vi "MultiScanDrift_dev_multiparam.vi"() -> ()   [LabVIEW 2014]
uses:
  shared/CorrelImages (SubVI)Single.vi
  <userlib>/Nanonis Prog Interface V5/Nanonis Prog Interface.lvlib
panel:
  out "size(s)":i32
  in  "max steps":i32
  in  "Lockin ON/OFF":bool
  in  "Multipass":bool=TRUE
  in  "Add":bool
  in  "end":sgl=1.0 format="%#_6p"
  in  "step":sgl=0.05 format="%#_6p"
  in  "start":sgl=-1.5 format="%#_6p"
  in  "create Range":bool
  in  "PLL ON/OFF":bool
  in  "ref bias":dbl=-0.0012 format="%#_6p"
  in  "ref setpoint":bool
  in  "DC On":bool=TRUE
  out "Y drift":i32
  out "X drift":i32
  out "DC active":bool
  in  "Drift correction Pixels":i32=128
  in  "Img Current":sgl=1e-10 format="%#_6p"
  in  "Img Bias (V) DC":sgl=1.0 format="%_2p"
  in  "Forward Speed":sgl=1.2e-09 format="%#_6p"
  in  "Backward Speed":sgl=8e-08 format="%#_6p"
  in  "Img Speed":sgl=4.5e-08 format="%#_6p"
  in  "Channel index (0-23)":u8(ring) items=["Current"=0, "Z (m)"=14]
  in  "Settling time (s)":dbl=0.7 format="%#_6p"
  in  "img bias":bool
  in  "img bias":dbl=-0.0012 format="%#_6p"
  in  "img delay (s)":u32=1
  out "Bias_mod":dbl format="%#_6p"
  in  "Bias_mod List":i32(listbox)
  in  "Const Height":bool
  in  "CurrentList":i32(listbox)
  in  "BiasList":i32(listbox)=35
  out "Current":dbl=5e-11 format="%#_6p"
  out "Bias":dbl=0.02 format="%#_6p"
  # "- Do Not Use This unless you are planning to change Lockin Amplitude for each bias. \n- This version will run experiments with parameters specified in each line."
  # "Turn continuous scan off\n zero tiplift is '0'"
  # "Multipass Windows \nneeds to be open\n and OFF"
  # "5"
  # "10"
  # "15"
  # "20"
  # "25"
  # "30"
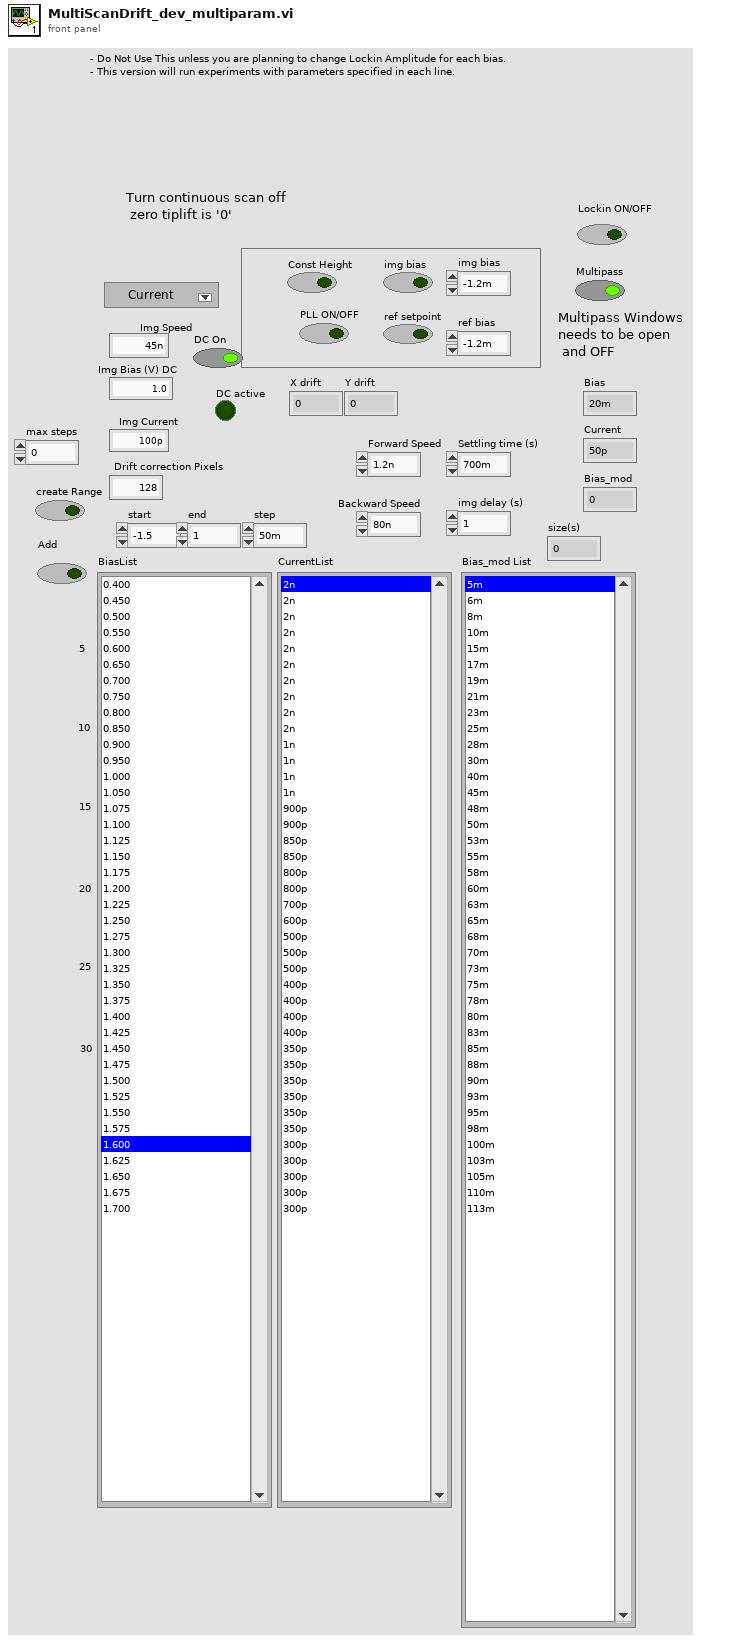
[diagram p1: front panel]
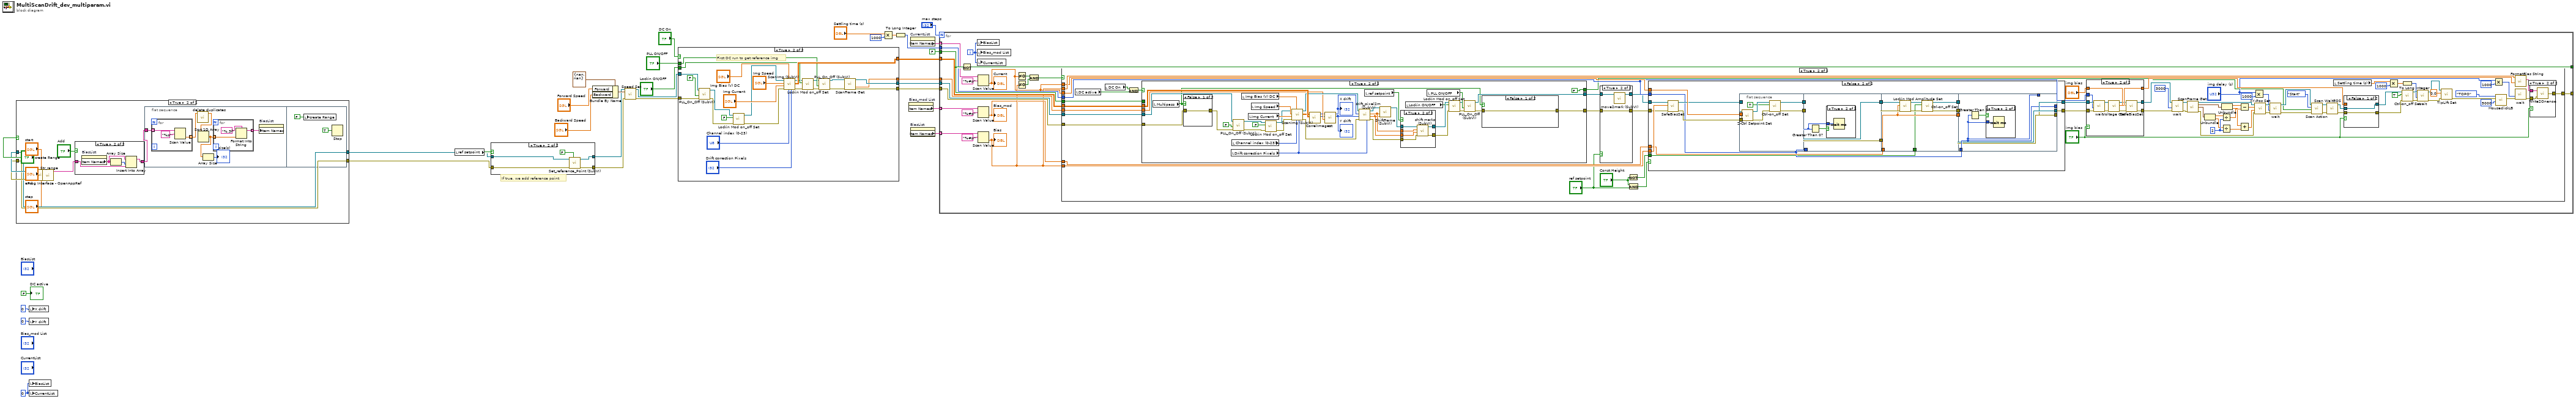
[diagram p0: block diagram]
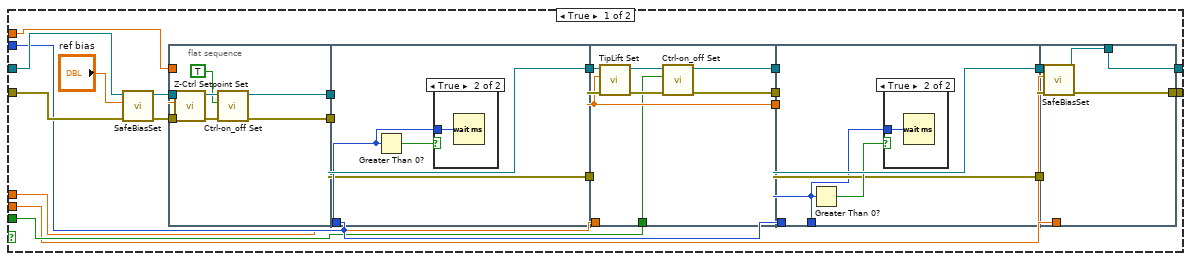
[diagram p4: hidden frame]
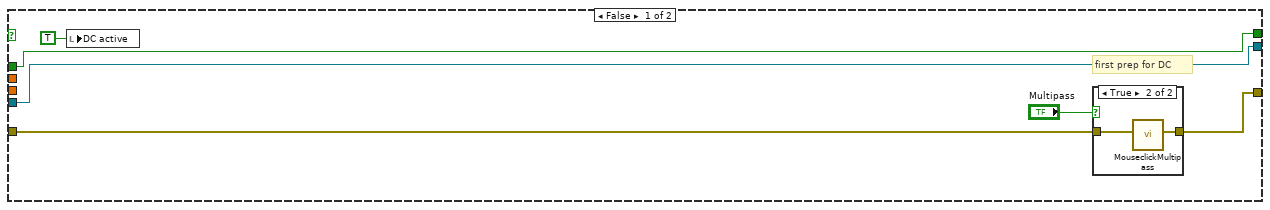
[diagram p10: hidden frame]
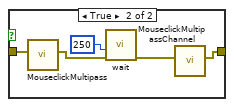
[diagram p13: hidden frame]
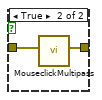
[diagram p14: hidden frame]
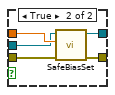
[diagram p15: hidden frame]
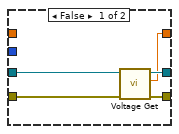
[diagram p16: hidden frame]
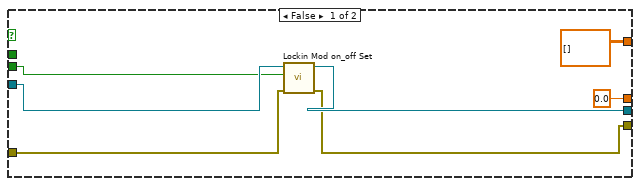
[diagram p20: hidden frame]
diagram:
  w34 = 0 ("BiasList")
  # "If true, we add reference point"
  n1 = local write "X drift"(0 ("X drift")) -> ()
  n2 = local write "Y drift"(0 ("Y drift")) -> ()
  n3 = local write "BiasList"(w34) -> ()
  n4 = local write "CurrentList"(w34) -> ()
  n5 = call <userlib>:"Prog Interface - OpenAppRef.vi"() -> ("Error out"=w9:errorcluster, "Application reference"=w10:refnum<vi>)  [unwired: 6 in]
  n6 = case shown="True" "create Range" {
    tunnel: w10 -> [w36 w44]
    tunnel: [w36 w44] -> w5
    tunnel: w9 -> [w35 w43]
    tunnel: [w35 w43] -> w7
    frame False {
    }
    frame True {
      n7 = call "Str_range.vi"("step"="step", "end"="end", "start"="start") -> ("Item Names"=w37:string[])  [unwired: 8 in]
      n8 = case shown="True" "Add" {
        tunnel: [w59 w61] -> w38
        tunnel: w37 -> [w59 w60]
        frame False {
        }
        frame True {
          n9 = property on="BiasList" class="LstBox (strict)"() -> ("Item Names"=w62:string[])  [unwired: 2 in, 2 out]
          n10 = Array Size(array=w62) -> (size(s)=w63:i32)
          n11 = Insert Into Array(array=w62, index=w63, new element=w60) -> (w61:string[])
        }
      }
      n12 = flat-sequence {
        tunnel: w38 -> [w50]
        frame #0 {
          n13 = for {
            tunnel: w50 -> [w56] mode=indexing
            tunnel: [w54] -> w46 mode=indexing
            n14 = Scan Value(string=w56, format string="%p") -> (value=w54:dbl)  [unwired: 1 in, 1 out]
          }
          n15 = call "delete duplicates.vi"("Array"=w46) -> ("Output array"=w45:dbl[])  [unwired: 10 in]
          n16 = Sort 1D Array(array=w45) -> (sorted array=w48:dbl[])
          n17 = Array Size(array=w48) -> (size(s)=→"size(s)":i32)
          n18 = for {
            tunnel: w48 -> [w53] mode=indexing
            tunnel: [w52] -> w49 mode=indexing
            n19 = Format Into String(format string="%.3f", w53) -> (resulting string=w52:string)  [unwired: 2 in, 1 out]
          }
          n20 = property on="BiasList" class="LstBox (strict)"("Item Names"=w49) -> ()  [unwired: 2 in, 2 out]
        }
        frame #1 {
          n21 = local write "create Range"(FALSE ("Range")) -> ()
          n22 = Stop(stop? (T)=TRUE) -> ()
        }
      }
    }
  }
  n23 = local read "ref setpoint"() -> (w8:bool)
  n24 = case shown="True" w8 {
    tunnel: w7 -> [w65 w69]
    tunnel: [w65 w68] -> w6
    tunnel: w5 -> [w64 w67]
    tunnel: [w64 w66] -> w4
    frame False {
    }
    frame True {
      n25 = call "Set_reference_Point (SubVI).vi"("Part of multigrid"=FALSE, "error in (no error)"=w69, "Application in"=w67) -> ("error out"=w68:errorcluster, "Application out"=w66:refnum<vi>)  [unwired: 7 in]
    }
  }
  n26 = Bundle By Name(cluster=cluster{"Forward":sgl, "Backward":sgl} {"Forward"=nan, "Backward"=nan} ("Speed (m/s)"), "Forward"="Forward Speed", "Backward"="Backward Speed") -> (w21:cluster{"Forward":sgl, "Backward":sgl})
  n27 = call <userlib>:"Speed Set.vi"("Application ref in"=w4, "Speed (m/s)"=w21, "error in (no error)"=w6) -> ("Application ref out"=w19:refnum<vi>, "error out"=w18:errorcluster)  [unwired: 11 in]
  n28 = case shown="True" "DC On" {
    tunnel: [w74 w91] -> w23
    tunnel: [w72 w90] -> w22
    tunnel: [dbl[][] [] ("Img") w98] -> w20
    tunnel: w19 -> [w75 w97]
    tunnel: w18 -> [w73 w96]
    tunnel: [sgl 0.0 ("Angle (deg)") w89] -> w13
    tunnel: "PLL ON/OFF" -> [_ w88]
    tunnel: "Lockin ON/OFF" -> [w71 w82]
    frame False {
      n29 = call <userlib>:"Lockin Mod on_off Set.vi"("Error in (no error)"=w73, "Lockin ON/OFF"=w71, "Application ref in"=w75) -> ("Error out"=w72:errorcluster, "Application ref out"=w74:refnum<vi>)  [unwired: 7 in]
    }
    frame True {
      # "First DC run to get reference img"
      n30 = call "PLL_On_Off (SubVI).vi"("error in (no error)"=w96, "Output ON/OFF (F=OFF)"=FALSE, "Application in"=w97) -> ("error out"=w85:errorcluster, "Application out"=w86:refnum<vi>)  [unwired: 7 in]
      n31 = call <userlib>:"Lockin Mod on_off Set.vi"("Error in (no error)"=w85, "Lockin ON/OFF"=FALSE, "Application ref in"=w86) -> ("Error out"=w84:errorcluster, "Application ref out"=w83:refnum<vi>)  [unwired: 7 in]
      n32 = call "ScanImg (SubVI).vi"("pixel"="Drift correction Pixels", "Channel index (0-23)"="Channel index (0-23)", "Bias (V)"="Img Bias (V) DC", "error in (no error)"=w84, "Current"="Img Current", "Img Speed"="Img Speed", "Application in"=w83) -> ("error out"=w79:errorcluster, "Img"=w98:dbl[][], "Application out"=w81:refnum<vi>)  [unwired: 2 in]
      n33 = call <userlib>:"Lockin Mod on_off Set.vi"("Error in (no error)"=w79, "Lockin ON/OFF"=w82, "Application ref in"=w81) -> ("Error out"=w78:errorcluster, "Application ref out"=w80:refnum<vi>)  [unwired: 7 in]
      n34 = call "PLL_On_Off (SubVI).vi"("error in (no error)"=w78, "Output ON/OFF (F=OFF)"=w88, "Application in"=w80) -> ("error out"=w92:errorcluster, "Application out"=w93:refnum<vi>)  [unwired: 7 in]
      n35 = call <userlib>:"ScanFrame Get.vi"("Application ref in"=w93, "error in (no error)"=w92) -> ("Application ref out"=w91:refnum<vi>, "Angle (deg)"=w89:sgl, "error out"=w90:errorcluster)  [unwired: 9 in, 2 out]
    }
  }
  n36 = Multiply(x="Settling time (s)", y=u32 1000) -> (x*y=w30:dbl)
  n37 = To Long Integer(number=w30) -> (32bit integer=w31:i32)
  n38 = property on="Bias_mod List" class="LstBox (strict)"() -> ("Item Names"=w2:string[])  [unwired: 2 in, 2 out]
  n39 = property on="CurrentList" class="LstBox (strict)"() -> ("Item Names"=w27:string[])  [unwired: 2 in, 2 out]
  n40 = property on="BiasList" class="LstBox (strict)"() -> ("Item Names"=w28:string[])  [unwired: 2 in, 2 out]
  n41 = for {
    N: "max steps" -> [_]
    tunnel: w28 -> [w118] mode=indexing
    tunnel: w23 -> [w120]
    tunnel: w22 -> [w119]
    tunnel: FALSE ("Direction: up/down (T=up)") -> [w122]
    tunnel: [w121] -> _
    tunnel: w31 -> [w114]
    tunnel: w20 -> [w113]
    tunnel: w13 -> [w112]
    tunnel: [w110] -> _
    tunnel: w27 -> [w107] mode=indexing
    tunnel: w2 -> [w106] mode=indexing
    i -> [w103]
    n42 = Not(x=w122) -> (.not. x?=w121:bool)
    n43 = local write "BiasList"(w103) -> ()
    n44 = local write "Bias_mod List"(w103) -> ()
    n45 = local write "CurrentList"(w103) -> ()
    n46 = Scan Value(string=w107, format string="%#p") -> (value=w105:dbl)  [unwired: 1 in, 1 out]
    "Current" <- w105
    n47 = Scan Value(string=w106, format string="%#p") -> (value=w104:dbl)  [unwired: 1 in, 1 out]
    "Bias_mod" <- w104
    n48 = Scan Value(string=w118, format string="%#p") -> (value=w111:dbl)  [unwired: 1 in, 1 out]
    "Bias" <- w111
    n49 = Not Equal To 0?(x=w105) -> (x != 0?=w117:bool)
    n50 = Not Equal To 0?(x=w111) -> (x != 0?=w116:bool)
    n51 = Compound Arithmetic op=AND(w117, w116) -> (w115:bool)
    n52 = case shown="True" w115 {
      tunnel: w122 -> [_ w176]
      tunnel: w111 -> [_ w202]
      tunnel: w120 -> [_ w181]
      tunnel: w119 -> [w124 w180]
      tunnel: w105 -> [_ w203]
      tunnel: w104 -> [_ w199]
      tunnel: w114 -> [_ w183]
      tunnel: w113 -> [_ w182]
      tunnel: w112 -> [_ w175]
      tunnel: w111 -> [_ w174]
      tunnel: w105 -> [_ w173]
      tunnel: [w124 w169] -> w110
      frame False {
      }
      frame True {
        w155 = 2
        n53 = local read "DC active"() -> (w179:bool)
        n54 = local read "DC On"() -> (w178:bool)
        n55 = And(x=w178, y=w179) -> (x .and. y?=w177:bool)
        n56 = case shown="True" w177 {
          tunnel: w182 -> [_ w357]
          tunnel: w181 -> [w314 w349]
          tunnel: w180 -> [w310 w338]
          tunnel: [w309 w334] -> w135
          tunnel: [w314 w348] -> w136
          tunnel: [w312 FALSE ("Direction: up/down (T=up)")] -> w140
          tunnel: w176 -> [w312 _]
          tunnel: w175 -> [_ w344]
          frame False {
            # "first prep for DC"
            n57 = local write "DC active"(TRUE ("DC active")) -> ()
            n58 = case shown="True" "Multipass" {
              tunnel: w310 -> [w315 w317]
              tunnel: [w315 w316] -> w309
              frame False {
              }
              frame True {
                n59 = call "MouseclickMultipass.vi"("error in (no error)"=w317) -> ("error out"=w316:errorcluster)  [unwired: 10 in]
              }
            }
          }
          frame True {
            n60 = local read "Multipass"() -> (w333:bool)
            n61 = case shown="False" w333 {
              tunnel: w338 -> [w372 w374]
              tunnel: [w372 w373] -> w337
              frame False {
              }
              frame True {
                n62 = call "MouseclickMultipass.vi"("error in (no error)"=w374) -> ("error out"=w373:errorcluster)  [unwired: 10 in]
              }
            }
            n63 = local read "Drift correction Pixels"() -> (w346:i32)
            n64 = local read "Channel index (0-23)"() -> (w352:u8)
            n65 = call "PLL_On_Off (SubVI).vi"("error in (no error)"=w337, "Output ON/OFF (F=OFF)"=FALSE, "Application in"=w349) -> ("error out"=w327:errorcluster, "Application out"=w325:refnum<vi>)  [unwired: 7 in]
            n66 = local read "Img Bias (V) DC"() -> (w353:sgl)
            n67 = local read "Img Current"() -> (w354:sgl)
            n68 = local read "Img Speed"() -> (w355:sgl)
            n69 = call <userlib>:"Lockin Mod on_off Set.vi"("Error in (no error)"=w327, "Lockin ON/OFF"=FALSE, "Application ref in"=w325) -> ("Error out"=w326:errorcluster, "Application ref out"=w324:refnum<vi>)  [unwired: 7 in]
            n70 = call "ScanImg (SubVI).vi"("pixel"=w346, "Channel index (0-23)"=w352, "Bias (V)"=w353, "error in (no error)"=w326, "Current"=w354, "Img Speed"=w355, "Application in"=w324) -> ("error out"=w336:errorcluster, "Img"=w356:dbl[][], "Application out"=w350:refnum<vi>)  [unwired: 2 in]
            n71 = call-poly "CorrelImages.vi"("Ref Array"=w357, "New Image"=w356) -> ("Y drift"=w341:i32, "X drift"=w343:i32)  [unwired: 6 in, 2 out]
            n72 = call "rot.vi"("angle"=w344, "y"=w341, "x"=w343) -> ("y'"=w340:i32, "x'"=w342:i32)  [unwired: 7 in]
            "X drift" <- w342
            "Y drift" <- w340
            n73 = call "drift_pixel2m (SubVI).vi"("Application in"=w350, "X drift"=w342, "Y drift"=w340, "error in"=w336, "Drift correction Pixels"=w346) -> ("Application out"=w351:refnum<vi>, "x drift"=w331:sgl, "y drift"=w330:sgl, "error out"=w329:errorcluster)  [unwired: 1 in]
            n74 = local read "ref setpoint"() -> (w332:bool)
            n75 = call "ShiftFrame (SubVI).vi"("Y shift"=w330, "X shift"=w331, "Application in"=w351) -> ("Application out"=w328:refnum<vi>)  [unwired: 8 in]
            n76 = case shown="True" w332 {
              tunnel: w331 -> [_ w365]
              tunnel: w330 -> [_ w364]
              tunnel: w329 -> [w358 w363]
              tunnel: [w358 w362] -> w320
              tunnel: w328 -> [w359 w361]
              tunnel: [w359 w360] -> w319
              frame False {
              }
              frame True {
                n77 = call "shift marks (SubVI).vi"("error in (no error)"=w363, "y"=w364, "x"=w365, "Application in"=w361) -> ("error out"=w362:errorcluster, "Application out"=w360:refnum<vi>)  [unwired: 6 in]
              }
            }
            n78 = local read "Lockin ON/OFF"() -> (w318:bool)
            n79 = local read "PLL ON/OFF"() -> (w339:bool)
            n80 = call <userlib>:"Lockin Mod on_off Set.vi"("Error in (no error)"=w320, "Lockin ON/OFF"=w318, "Application ref in"=w319) -> ("Error out"=w321:errorcluster, "Application ref out"=w322:refnum<vi>)  [unwired: 7 in]
            n81 = call "PLL_On_Off (SubVI).vi"("error in (no error)"=w321, "Output ON/OFF (F=OFF)"=w339, "Application in"=w322) -> ("error out"=w335:errorcluster, "Application out"=w348:refnum<vi>)  [unwired: 7 in]
            n82 = case shown="False" w333 {
              tunnel: w335 -> [w366 w371]
              tunnel: [w366 w370] -> w334
              frame False {
              }
              frame True {
                n83 = call "MouseclickMultipass.vi"("error in (no error)"=w371) -> ("error out"=w369:errorcluster)  [unwired: 10 in]
                n84 = call "wait.vi"("error in"=w369, "milliseconds to wait"=u32 250) -> ("error out"=w368:errorcluster)  [unwired: 8 in, 1 out]
                n85 = call "MouseclickMultipassChannel.vi"("error in (no error)"=w368) -> ("error out"=w370:errorcluster)  [unwired: 10 in]
              }
            }
          }
        }
        n86 = case shown="True" "ref setpoint" {
          tunnel: w136 -> [w205 w208]
          tunnel: w135 -> [w204 w207]
          tunnel: [w204 w207] -> w133
          tunnel: [w205 w206] -> w134
          frame False {
          }
          frame True {
            n87 = call "move2mark (SubVI).vi"("Application in"=w208) -> ("Application out"=w206:refnum<vi>)  [unwired: 10 in]
          }
        }
        n88 = Not(x="Const Height") -> (.not. x?=w201:bool)
        n89 = And(x="Const Height", y="ref setpoint") -> (x .and. y?=w167:bool)
        n90 = case shown="False" w167 {
          tunnel: w203 -> [w216 w268]
          tunnel: w202 -> [w211 w278]
          tunnel: w201 -> [w212 w263]
          tunnel: w199 -> [w213 w265]
          tunnel: [w210 w262] -> w196
          tunnel: [w209 w261] -> w195
          tunnel: w183 -> [w217 w264]
          tunnel: w133 -> [w227 w277]
          tunnel: w134 -> [w228 w276]
          frame True {
            n91 = call "SafeBiasSet.vi"("Application ref in"=w228, "Bias (V)"="ref bias", "error in (no error)"=w227) -> ("Application ref out"=w215:refnum<vi>, "Error out"=w214:errorcluster)  [unwired: 6 in]
            n92 = flat-sequence {
              tunnel: [w236] -> w226
              tunnel: [w233] -> w225
              tunnel: w216 -> [w232]
              tunnel: w215 -> [w231]
              tunnel: w214 -> [w230]
              tunnel: w226 -> [w241]
              tunnel: [w241] -> w224
              tunnel: w217 -> [w239]
              tunnel: [w238] -> w223
              tunnel: w225 -> [w238]
              tunnel: w224 -> [w250]
              tunnel: [w248] -> w222
              tunnel: [w244] -> w221
              tunnel: w223 -> [w247]
              tunnel: [w245] -> w220
              tunnel: w213 -> [w244]
              tunnel: w212 -> [w243]
              tunnel: w222 -> [w254]
              tunnel: [w251] -> _
              tunnel: w221 -> [_]
              tunnel: [w254] -> w219
              tunnel: [w252] -> w218
              tunnel: w220 -> [w252]
              tunnel: w217 -> [w251]
              tunnel: [w259] -> w210
              tunnel: w219 -> [w260]
              tunnel: w218 -> [w258]
              tunnel: [w257] -> w209
              tunnel: w211 -> [w256]
              frame #0 {
                n93 = call <userlib>:"Z-Ctrl Setpoint Set.vi"("error in (no error)"=w230, "Z Controller setpoint"=w232, "Application ref in"=w231) -> ("error out"=w234:errorcluster, "Application ref out"=w237:refnum<vi>)  [unwired: 7 in]
                n94 = call <userlib>:"Ctrl-on_off Set.vi"("error in (no error)"=w234, "Z Controller ON/OFF"=TRUE, "Application ref in"=w237) -> ("error out"=w233:errorcluster, "Application ref out"=w236:refnum<vi>)  [unwired: 7 in]
              }
              frame #1 {
                n95 = Greater Than 0?(x=w239) -> (x > 0?=w240:bool)
                n96 = case shown="True" w240 {
                  tunnel: w239 -> [_ w242]
                  frame False {
                  }
                  frame True {
                    n97 = Wait (ms)(milliseconds to wait=w242) -> ()  [unwired: 1 out]
                  }
                }
              }
              frame #2 {
                n98 = call <userlib>:"TipLift Set.vi"("error in (no error)"=w247, "TipLift (m)"=w244, "Application ref in"=w250) -> ("error out"=w246:errorcluster, "Application ref out"=w249:refnum<vi>)  [unwired: 7 in]
                n99 = call <userlib>:"Ctrl-on_off Set.vi"("error in (no error)"=w246, "Z Controller ON/OFF"=w243, "Application ref in"=w249) -> ("error out"=w245:errorcluster, "Application ref out"=w248:refnum<vi>)  [unwired: 7 in]
              }
              frame #3 {
                n100 = Greater Than 0?(x=w251) -> (x > 0?=w253:bool)
                n101 = case shown="True" w253 {
                  tunnel: w251 -> [_ w255]
                  frame False {
                  }
                  frame True {
                    n102 = Wait (ms)(milliseconds to wait=w255) -> ()  [unwired: 1 out]
                  }
                }
              }
              frame #4 {
                n103 = call "SafeBiasSet.vi"("Application ref in"=w260, "Bias (V)"=w256, "error in (no error)"=w258) -> ("Application ref out"=w259:refnum<vi>, "Error out"=w257:errorcluster)  [unwired: 6 in]
              }
            }
          }
          frame False {
            n104 = call "SafeBiasSet.vi"("Application ref in"=w276, "Bias (V)"=w278, "error in (no error)"=w277) -> ("Application ref out"=w267:refnum<vi>, "Error out"=w266:errorcluster)  [unwired: 6 in]
            n105 = flat-sequence {
              tunnel: [w285] -> w275
              tunnel: [w282] -> w274
              tunnel: w268 -> [w281]
              tunnel: w267 -> [w280]
              tunnel: w266 -> [w279]
              tunnel: w275 -> [w290]
              tunnel: [w290] -> w273
              tunnel: w264 -> [w288]
              tunnel: [w287] -> w272
              tunnel: w274 -> [w287]
              tunnel: w273 -> [w299]
              tunnel: [w297] -> w271
              tunnel: [w293] -> w270
              tunnel: w272 -> [w296]
              tunnel: [w294] -> w269
              tunnel: w265 -> [w293]
              tunnel: w263 -> [w292]
              tunnel: w264 -> [w302]
              tunnel: [w302] -> _
              tunnel: w269 -> [w300]
              tunnel: w270 -> [_]
              tunnel: [w302] -> _
              tunnel: w271 -> [w301]
              tunnel: [w301] -> w262
              tunnel: [w300] -> w261
              frame #0 {
                n106 = call <userlib>:"Z-Ctrl Setpoint Set.vi"("error in (no error)"=w279, "Z Controller setpoint"=w281, "Application ref in"=w280) -> ("error out"=w283:errorcluster, "Application ref out"=w286:refnum<vi>)  [unwired: 7 in]
                n107 = call <userlib>:"Ctrl-on_off Set.vi"("error in (no error)"=w283, "Z Controller ON/OFF"=TRUE, "Application ref in"=w286) -> ("error out"=w282:errorcluster, "Application ref out"=w285:refnum<vi>)  [unwired: 7 in]
              }
              frame #1 {
                n108 = Greater Than 0?(x=w288) -> (x > 0?=w289:bool)
                n109 = case shown="True" w289 {
                  tunnel: w288 -> [_ w291]
                  frame False {
                  }
                  frame True {
                    n110 = Wait (ms)(milliseconds to wait=w291) -> ()  [unwired: 1 out]
                  }
                }
              }
              frame #2 {
                n111 = call <userlib>:"Lockin Mod Amplitude Set.vi"("Error in (no error)"=w296, "Amplitude (mod. signal unit)"=w293, "Application ref in"=w299) -> ("Error out"=w295:errorcluster, "Application ref out"=w298:refnum<vi>)  [unwired: 7 in]
                n112 = call <userlib>:"Ctrl-on_off Set.vi"("error in (no error)"=w295, "Z Controller ON/OFF"=w292, "Application ref in"=w298) -> ("error out"=w294:errorcluster, "Application ref out"=w297:refnum<vi>)  [unwired: 7 in]
              }
              frame #3 {
                n113 = Greater Than 0?(x=w302) -> (x > 0?=w303:bool)
                n114 = case shown="True" w303 {
                  tunnel: w302 -> [_ w304]
                  frame False {
                  }
                  frame True {
                    n115 = Wait (ms)(milliseconds to wait=w304) -> ()  [unwired: 1 out]
                  }
                }
              }
            }
          }
        }
        n116 = case shown="True" "img bias" {
          tunnel: w196 -> [w386 w393]
          tunnel: [w385 w389] -> w138
          tunnel: w195 -> [w382 w396]
          tunnel: [w383 w390] -> w139
          tunnel: "img bias" -> [_ w391]
          tunnel: [w384 w397] -> w193
          tunnel: w183 -> [_ w392]
          frame False {
            n117 = call <userlib>:"Voltage Get.vi"("error in (no error)"=w382, "Application ref in"=w386) -> ("error out"=w383:errorcluster, "Bias (V)"=w384:sgl, "Application ref out"=w385:refnum<vi>)  [unwired: 7 in]
          }
          frame True {
            n118 = call "wait.vi"("error in"=w396, "milliseconds to wait"=w392, "application reference in"=w393) -> ("error out"=w395:errorcluster, "application reference out"=w394:refnum<vi>)  [unwired: 7 in]
            n119 = call <userlib>:"Voltage Get.vi"("error in (no error)"=w395, "Application ref in"=w394) -> ("error out"=w387:errorcluster, "Bias (V)"=w397:sgl, "Application ref out"=w388:refnum<vi>)  [unwired: 7 in]
            n120 = call "SafeBiasSet.vi"("Application ref in"=w388, "Bias (V)"=w391, "error in (no error)"=w387) -> ("Application ref out"=w389:refnum<vi>, "Error out"=w390:errorcluster)  [unwired: 6 in]
          }
        }
        n121 = call "wait.vi"("error in"=w139, "milliseconds to wait"=u32 3000 ("y"), "application reference in"=w138) -> ("error out"=w147:errorcluster, "application reference out"=w146:refnum<vi>)  [unwired: 7 in]
        n122 = call <userlib>:"ScanFrame Get.vi"("Application ref in"=w146, "error in (no error)"=w147) -> ("Application ref out"=w166:refnum<vi>, "Center coordinates (m)"=w150:cluster{"Xc":sgl, "Yc":sgl}, "Size (m)"=w151:cluster{"Width":sgl, "Height":sgl}, "error out"=w165:errorcluster)  [unwired: 9 in, 1 out]
        n123 = Unbundle(w151) -> ("Width"=w153:sgl, "Height"=w154:sgl)
        n124 = Divide(x=w153, y=w155) -> (x/y=w157:sgl)
        n125 = Divide(x=w154, y=w155) -> (x/y=w156:sgl)
        n126 = Unbundle(w150) -> ("Xc"=w158:sgl, "Yc"=w152:sgl)
        n127 = Subtract(x=w158, y=w157) -> (x-y=w159:sgl)
        n128 = Add(x=w152, y=w156) -> (x+y=w160:sgl)
        n129 = Multiply(x="img delay (s)", y=u32 1000) -> (x*y=w162:u32)
        n130 = call <userlib>:"XY-Pos Set.vi"("error in (no error)"=w165, "Y (m)"=w160, "X (m)"=w159, "Application ref in"=w166) -> ("error out"=w164:errorcluster, "Application ref out"=w163:refnum<vi>)  [unwired: 4 in]
        n131 = call "wait.vi"("error in"=w164, "milliseconds to wait"=w162, "application reference in"=w163) -> ("error out"=w144:errorcluster, "application reference out"=w145:refnum<vi>)  [unwired: 7 in]
        n132 = call <userlib>:"Scan Action.vi"("error in (no error)"=w144, "Direction: up/down (T=up)"=w140, "Scan action (Start)"=enum16{"Start", "Stop", "Pause", "Resume"}."Start", "Application ref in"=w145) -> ("error out"=w142:errorcluster, "Application ref out"=w143:refnum<vi>)  [unwired: 5 in]
        n133 = call <userlib>:"Scan WaitEOS.vi"("error in (no error)"=w142, "Application ref in"=w143) -> ("error out"=w191:errorcluster, "Application ref out"=w192:refnum<vi>)  [unwired: 5 in, 2 out]
        n134 = local read "Settling time (s)"() -> (w126:dbl)
        n135 = case shown="False" "img bias" {
          tunnel: w192 -> [w376 w377]
          tunnel: [w376 w380] -> w190
          tunnel: [w375 w381] -> w189
          tunnel: w191 -> [w375 w379]
          tunnel: w193 -> [_ w378]
          frame False {
          }
          frame True {
            n136 = call "SafeBiasSet.vi"("Application ref in"=w377, "Bias (V)"=w378, "error in (no error)"=w379) -> ("Application ref out"=w380:refnum<vi>, "Error out"=w381:errorcluster)  [unwired: 6 in]
          }
        }
        n137 = Multiply(x=w126, y=u32 1000) -> (x*y=w127:dbl)
        n138 = To Long Integer(number=w127) -> (32bit integer=w125:i32)
        n139 = call <userlib>:"Ctrl-on_off Set.vi"("error in (no error)"=w189, "Z Controller ON/OFF"=TRUE, "Application ref in"=w190) -> ("error out"=w132:errorcluster, "Application ref out"=w130:refnum<vi>)  [unwired: 7 in]
        n140 = call "wait.vi"("error in"=w132, "milliseconds to wait"=w125, "application reference in"=w130) -> ("error out"=w131:errorcluster, "application reference out"=w129:refnum<vi>)  [unwired: 7 in]
        n141 = call <userlib>:"TipLift Set.vi"("error in (no error)"=w131, "TipLift (m)"=sgl 0.0, "Application ref in"=w129) -> ("error out"=w198:errorcluster)  [unwired: 7 in, 1 out]
        n142 = Multiply(x="img delay (s)", y=u32 1000) -> (x*y=w185:u32)
        n143 = call "MouseclickLB.vi"("nMilliseconds"=5000, "error in (no error)"=w198, "Click"=enum16{"Header", "TOPO", "STS", "GRID"}."TOPO") -> ("error out"=w184:errorcluster)  [unwired: 8 in]
        n144 = call "FormatBias String.vi"("current"=w173, "bias"=w174) -> ("resulting string"=w170:string)  [unwired: 9 in]
        n145 = call "wait.vi"("error in"=w184, "milliseconds to wait"=w185) -> ("error out"=w171:errorcluster)  [unwired: 8 in, 1 out]
        n146 = case shown="True" "img bias" {
          tunnel: w171 -> [w305 w308]
          tunnel: w170 -> [_ w307]
          tunnel: [w305 w306] -> w169
          frame False {
          }
          frame True {
            n147 = call "Write2Onenoe.vi"("error in (no error)"=w308, "strSendText"=w307) -> ("error out"=w306:errorcluster)
          }
        }
      }
    }
  }
  "DC active" <- FALSE ("DC active")
